vi "Practica3_Secuencia.vi"() -> ()   [LabVIEW 2022 SP3]
panel:
  out "Divide A/B":dbl(slide) scale=-25.0..25.0
  out "Resta A - B":dbl
  out "Multiplica A x B":dbl(knob) scale=0.0..50.0
  out "Suma A + B":dbl(knob) scale=0.0..50.0
  out "A<B":bool
  out "A>B":bool
  out "A=B":bool
  in  "Variable B":dbl(knob) scale=0.0..10.0
  in  "Variable A":dbl(knob) scale=0.0..10.0
  # "Anahí Montserrat Vázquez Padilla \nPráctica 04: Secuencia \n30/01/2024"
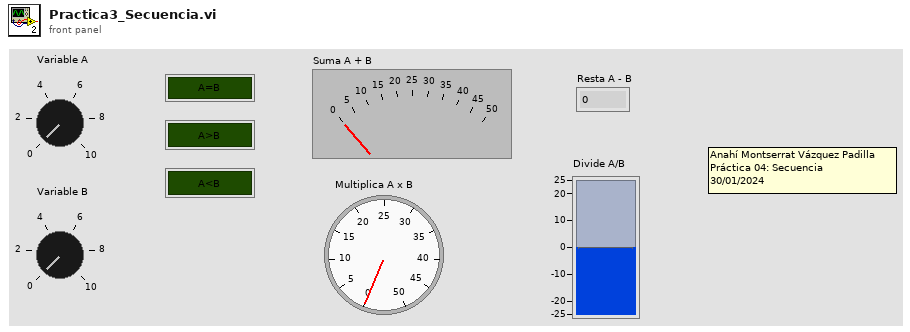
[diagram p1: front panel]
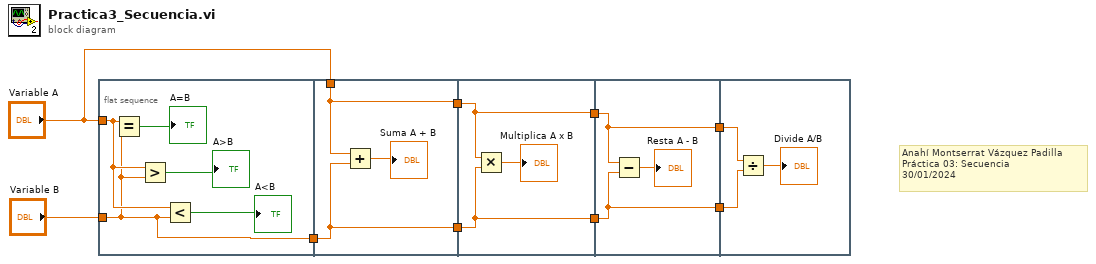
[diagram p0: block diagram]
diagram:
  # "Anahí Montserrat Vázquez Padilla \nPráctica 03: Secuencia \n30/01/2024"
  n1 = flat-sequence {
    tunnel: "Variable A" -> [w14]
    tunnel: "Variable B" -> [w10]
    tunnel: [w10] -> w7
    tunnel: "Variable A" -> [w16]
    tunnel: w7 -> [w15]
    tunnel: [w16] -> w6
    tunnel: [w15] -> w5
    tunnel: w6 -> [w19]
    tunnel: w5 -> [w18]
    tunnel: [w19] -> w4
    tunnel: [w18] -> w3
    tunnel: w4 -> [w22]
    tunnel: w3 -> [w21]
    tunnel: [w22] -> w2
    tunnel: [w21] -> w1
    tunnel: w2 -> [w26]
    tunnel: w1 -> [w25]
    frame #0 {
      n2 = Equal?(x=w14, y=w10) -> (x = y?=→"A=B":bool)
      n3 = Greater?(x=w14, y=w10) -> (0:→"A>B":bool)
      n4 = Less?(x=w14, y=w10) -> (x < y?=→"A<B":bool)
    }
    frame #1 {
      n5 = Add(x=w16, y=w15) -> (x+y=→"Suma A + B":dbl)
    }
    frame #2 {
      n6 = Multiply(x=w19, y=w18) -> (x*y=→"Multiplica A x B":dbl)
    }
    frame #3 {
      n7 = Subtract(x=w22, y=w21) -> (x-y=→"Resta A - B":dbl)
    }
    frame #4 {
      n8 = Divide(x=w26, y=w25) -> (x/y=→"Divide A/B":dbl)
    }
  }
